vi "Set Step Name.vi"(8 "error in (no error)":errorcluster, 10 "Standard":string, 11 "Input Power Measurement in":refnum<class "Input Power Measurement.lvclass">) -> (0 "error out":errorcluster, 2 "Default Step":string, 3 "Input Power Measurement out":refnum<class "Input Power Measurement.lvclass">)   [LabVIEW 2018, in "Input Power Measurement.lvlib" / "Input Power Measurement.lvclass"]
uses:
  Input Power Measurement.lvclass
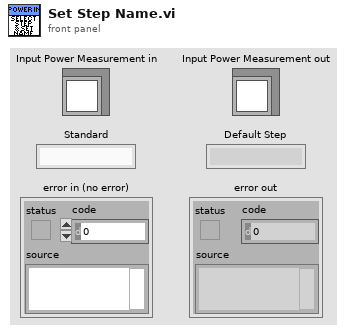
[diagram p1: front panel]
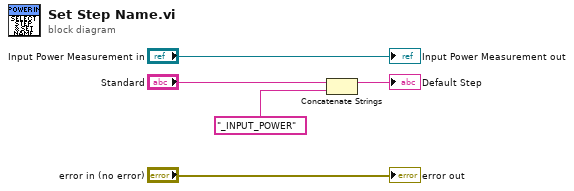
[diagram p0: block diagram]
diagram:
  n1 = Concatenate Strings("Standard", "_INPUT_POWER" ("string")) -> (→"Default Step":string)
  "error out" <- "error in (no error)"
  "Input Power Measurement out" <- "Input Power Measurement in"
